vi "AFCtoPreformTiming.vi"(11 "Input Trigger Data":T3) -> (3 "Output Trigger Data":T3)   [LabVIEW 2016]
uses:
  Ctrl_Signal.ctl
  Ctrl_Signal_Map.ctl
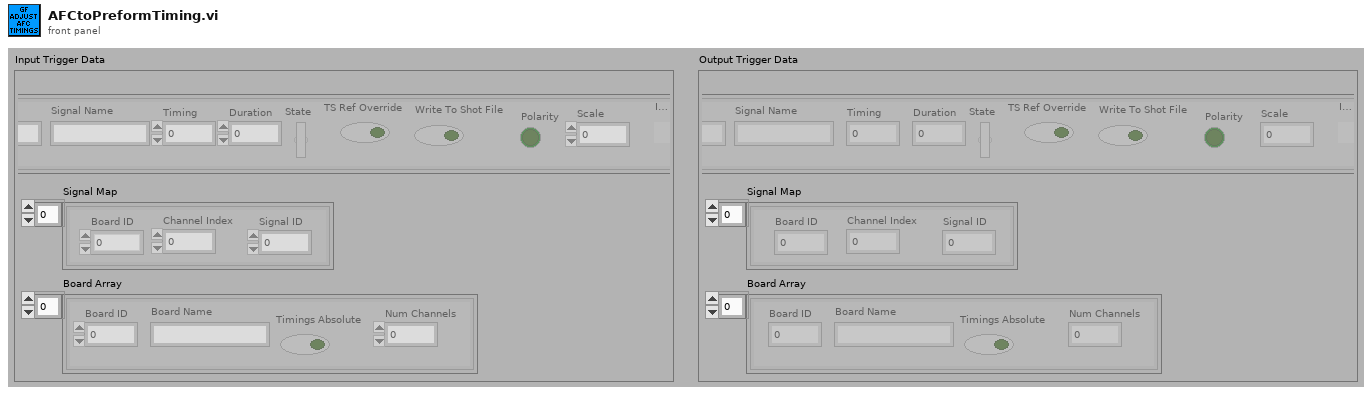
[diagram p1: front panel]
types:
  T1 = typedef "Ctrl_Signal.ctl" = cluster{"Signal Name":string, "Timing":dbl, "Duration":dbl, "State":bool, "TS Ref Override":bool, "Write To Shot File":bool, "Polarity":bool, "Signal ID":dbl, "Scale":dbl, "IsDelay":bool}
  T2 = typedef "Ctrl_Signal_Map.ctl" = cluster{"Channel Index":dbl, "Board ID":dbl, "Signal ID":dbl}
  T3 = cluster{"Signal Array":T1[], "Signal Map":T2[], "Board Array":cluster{"Board ID":dbl, "Board Name":string, "Timings Absolute":bool, "Num Channels":dbl}[]}
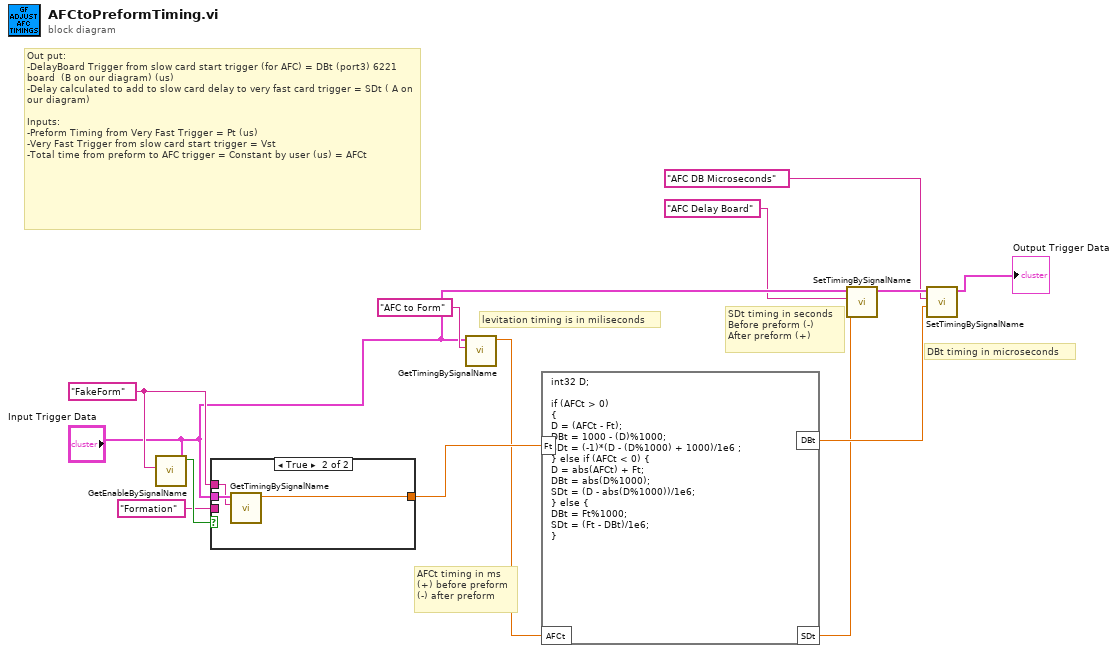
[diagram p0: block diagram]
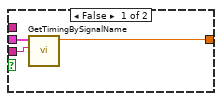
[diagram p2: hidden frame]
diagram:
  w12 = "FakeForm" ("Signal Name")
  # "AFCt timing in ms\n(+) before preform\n(-) after preform"
  # "SDt timing in seconds\nBefore preform (-) \nAfter preform (+)"
  # "DBt timing in microseconds"
  # "levitation timing is in miliseconds"
  # "Out put: \n-DelayBoard Trigger from slow card start trigger (for AFC) = DBt (port3) 6221 board  (B on our diagram) (us)\n-Delay calculated to add to slow card delay to very fast card trigger = SDt ( A on our diagram)\n\nInputs:\n-Preform Timing from Very Fast Trigger = Pt (us)\n-Very Fast Trigger from slow card start trigger = Vst\n-Total time from preform to AFC trigger = Constant by user (us) = AFCt"
  n1 = call "GetEnableBySignalName.vi"("Signal Name"=w12, "Trigger Data"="Input Trigger Data") -> ("Signal Enabled"=w13:bool)  [unwired: 9 in]
  n2 = case shown="True" w13 {
    tunnel: "Input Trigger Data" -> [w16 w19]
    tunnel: w12 -> [_ w18]
    tunnel: "Formation" ("Signal Name") -> [w15 _]
    tunnel: [w14 w17] -> w4
    frame False {
      n3 = call "GetTimingBySignalName.vi"("Signal Name"=w15, "Trigger Data"=w16) -> ("Timing"=w14:dbl)  [unwired: 9 in]
    }
    frame True {
      n4 = call "GetTimingBySignalName.vi"("Signal Name"=w18, "Trigger Data"=w19) -> ("Timing"=w17:dbl)  [unwired: 9 in]
    }
  }
  n5 = call "GetTimingBySignalName.vi"("Signal Name"="AFC to Form", "Trigger Data"="Input Trigger Data") -> ("Timing"=w3:dbl)  [unwired: 9 in]
  n6 = formula code="int32 D;\n\nif (AFCt > 0)\n{\nD = (AFCt - Ft);\nDBt = 1000 - (D)%1000;\nSDt = (-1)*(D - (D%1000) + 1000)/1e6 ;\n} else if (AFCt < 0) {\nD = abs(AFCt) + Ft;\nDBt = abs(D%1000);\nSDt = (D - abs(D%1000))/1e6;\n} else {\nDBt = Ft%1000;\nSDt = (Ft - DBt)/1e6;\n}"("Ft"=w4, "AFCt"=w3) -> ("DBt"=w2:dbl, "SDt"=w1:dbl)
  n7 = call "SetTimingBySignalName.vi"("Timing"=w1, "Signal Name"="AFC Delay Board", "Trigger Data Input"="Input Trigger Data") -> ("Trigger Data Output"=w8:T3)  [unwired: 8 in]
  n8 = call "SetTimingBySignalName.vi"("Timing"=w2, "Signal Name"="AFC DB Microseconds", "Trigger Data Input"=w8) -> ("Trigger Data Output"=→"Output Trigger Data":T3)  [unwired: 8 in]
